vi "Construct.vi"(8 "error in (no error)":errorcluster, 11 "RT FIFO I64 Notifier in":refnum<class "RT FIFO I64 Notifier.lvclass">) -> (0 "error out":errorcluster, 3 "RT FIFO I64 Notifier out":refnum<class "RT FIFO I64 Notifier.lvclass">)   [LabVIEW 2024, in "RT FIFO I64 Notifier.lvclass"]
uses:
  RT FIFO I64 Notifier.lvclass
  RT FIFO I64 Notifier.lvclass/RT FIFO I64 Notifier.ctl
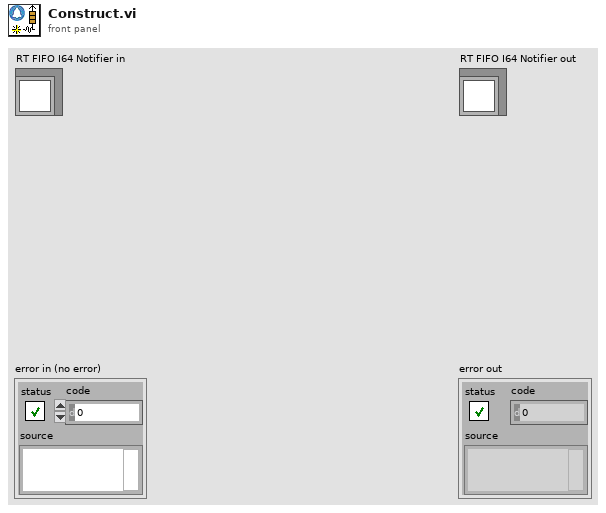
[diagram p1: front panel]
types:
  T1 = cluster{"read mode":enum16{"polling", "blocking"}, "write mode":enum16{"polling", "blocking"}}
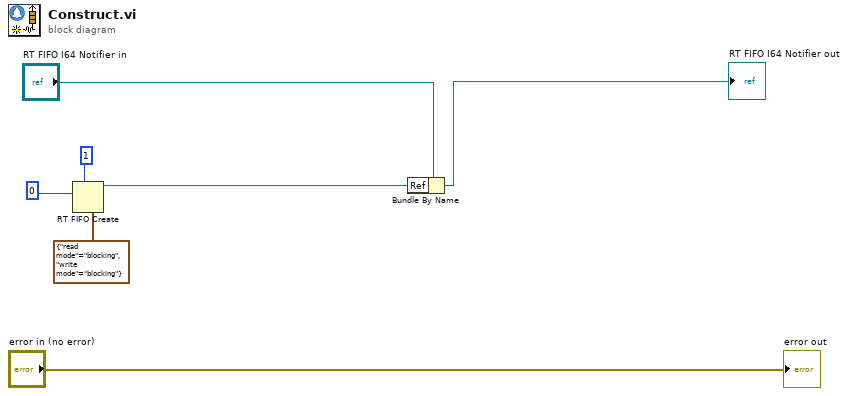
[diagram p0: block diagram]
diagram:
  n1 = RT FIFO Create(1:i64 0, 4:u32 1 ("size (10)"), 7:T1 {"read mode"=enum."blocking", "write mode"=enum."blocking"} ("r/w modes (polling,polling)")) -> (8:w1:refnum<k33>)  [unwired: 5 in, 2 out]
  n2 = Bundle By Name(cluster="RT FIFO I64 Notifier in", "Ref"=w1) -> (→"RT FIFO I64 Notifier out":refnum<class "RT FIFO I64 Notifier.lvclass">)
  "error out" <- "error in (no error)"
